vi "MOTOR CONTROL WITH PID AE.vi"(1 "Yaw":dbl, 2 "Speed":dbl, 3 "Direction":T1, 4 "AE Mode":T2) -> (0 "Speed & distance":T3)   [LabVIEW 2018]
uses:
  MOTOR CONTROL WITH PID AE DATA MODE TYPE DEF.ctl
  MOTOR CONTROL WITH PID AE DIRECTION TYPE DEF.ctl
  <vilib>/Studica/Studica Toolkit/Background/Mxp Selection.ctl
  <vilib>/addons/control/pid/pid.llb/PID (DBL).vi
  <vilib>/addons/control/pid/NI_PID_pid.lvlib
panel:
  out "Vx":dbl
  in  "error in (no error)":errorcluster
  out "M2":dbl
  out "M1":dbl
  out "M0":dbl
  out "S2":dbl
  out "S1":dbl
  out "error out":errorcluster
  out "S0":dbl
  out "M2 Distance":dbl
  out "M1 Distance":dbl
  out "M0 Distance":dbl
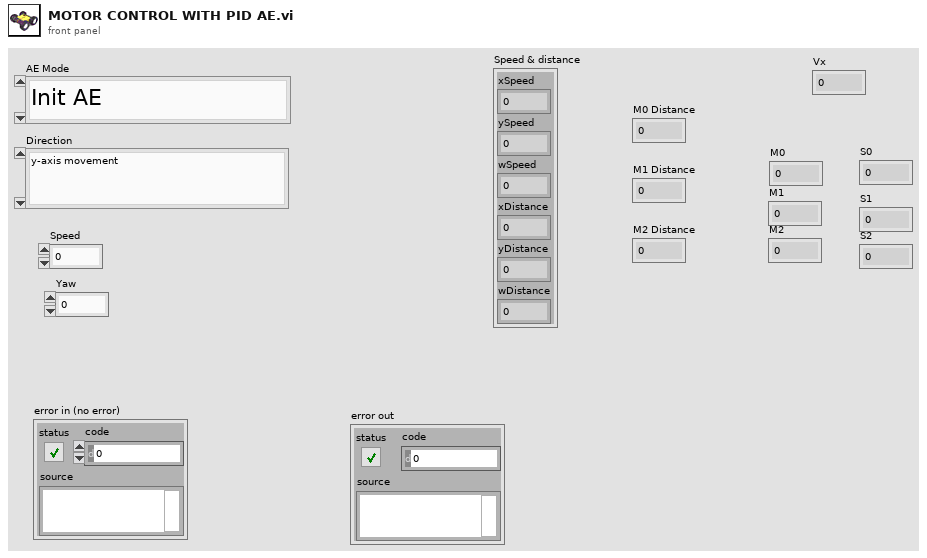
[diagram p1: front panel]
types:
  T1 = typedef "MOTOR CONTROL WITH PID AE DIRECTION TYPE DEF.ctl" = enum16{"y-axis movement", "x-axis movement", "rotation", "stop", "reset encoders"}
  T2 = typedef "MOTOR CONTROL WITH PID AE DATA MODE TYPE DEF.ctl" = enum16{"Init AE", "Write to AE", "Read from AE"}
  T3 = cluster{"xSpeed":dbl, "ySpeed":dbl, "wSpeed":dbl, "xDistance":dbl, "yDistance":dbl, "wDistance":dbl}
  T4 = cluster{"proportional gain (Kc)":dbl, "integral time (Ti, min)":dbl, "derivative time (Td, min)":dbl}
  T5 = typedef "Mxp Selection.ctl" = enum16{"MXP A", "MXP B"}
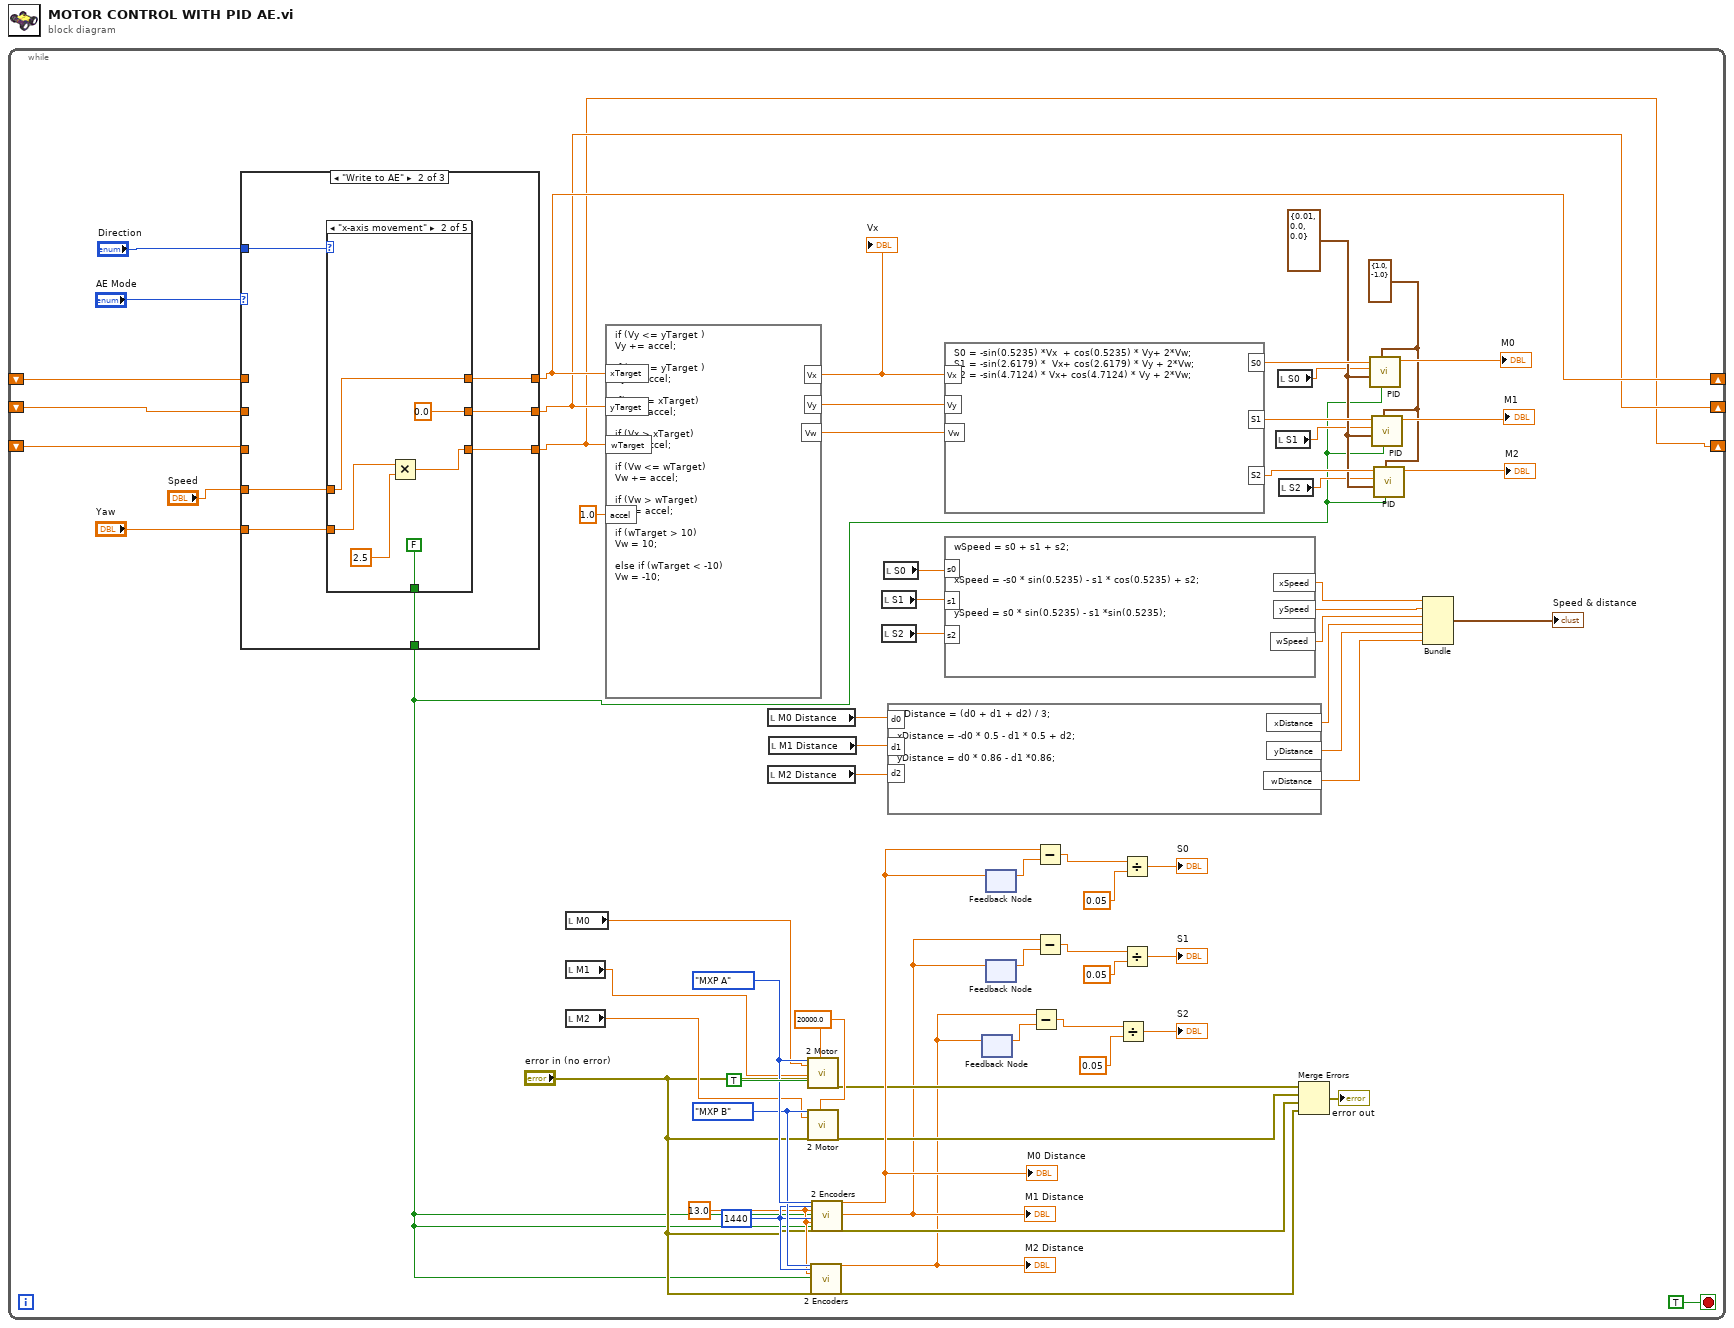
[diagram p0: block diagram]
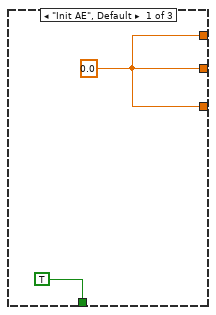
[diagram p2: hidden frame]
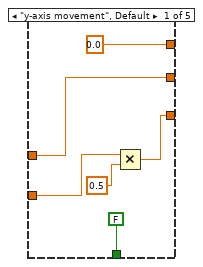
[diagram p3: hidden frame]
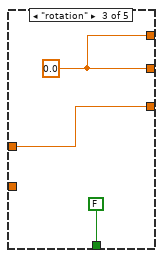
[diagram p4: hidden frame]
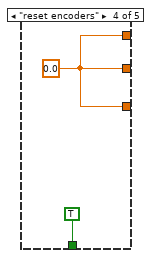
[diagram p5: hidden frame]
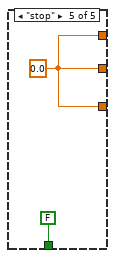
[diagram p6: hidden frame]
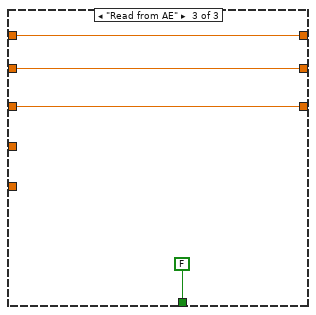
[diagram p7: hidden frame]
diagram:
  n1 = while {
    shift-right: [w9] -> _
    shift-left: _ -> [w12]
    shift-right: [w8] -> _
    shift-left: _ -> [w11]
    shift-right: [w7] -> _
    shift-left: _ -> [w10]
    stop <- TRUE stop-if-true
    w17 = T4 {"proportional gain (Kc)"=0.01, "integral time (Ti, min)"=0.0, "derivative time (Td, min)"=0.0} ("PID gains")
    w16 = cluster{"output high":dbl, "output low":dbl} {"output high"=1.0, "output low"=-1.0} ("output range")
    w65 = 13.0 ("Wheel Diameter M0 (inches)")
    w66 = u32 1440 ("Ticks Per Rev M0")
    w70 = 20000.0 ("Frequency [Hz]")
    w68 = Mxp_Selection."MXP A" ("Mxp Side")
    w67 = Mxp_Selection."MXP B" ("Mxp Side")
    n2 = case shown="\"Write to AE\"" "AE Mode" {
      tunnel: "Direction" -> [_ w79 _]
      tunnel: "Speed" -> [_ w78 _]
      tunnel: "Yaw" -> [_ w77 _]
      tunnel: [w72 w76 w101] -> w9
      tunnel: [w72 w75 w99] -> w7
      tunnel: [w72 w74 w100] -> w8
      tunnel: w12 -> [_ _ w101]
      tunnel: w11 -> [_ _ w100]
      tunnel: w10 -> [_ _ w99]
      tunnel: [TRUE w73 FALSE] -> w6
      frame "Init AE", Default {
        w72 = 0.0 ("input variable")
      }
      frame "Write to AE" {
        n3 = case shown="\"x-axis movement\"" w79 {
          tunnel: w78 -> [w85 w91 w94 _ _]
          tunnel: w77 -> [w82 w88 _ _ _]
          tunnel: [0.0 ("Speed") w91 w93 w96 w98] -> w76
          tunnel: [w81 w86 w94 w96 w98] -> w75
          tunnel: [w85 0.0 ("input variable") w93 w96 w98] -> w74
          tunnel: [FALSE FALSE FALSE TRUE FALSE] -> w73
          frame "y-axis movement", Default {
            n4 = Multiply(x=w82, y=0.5) -> (x*y=w81:dbl)
          }
          frame "x-axis movement" {
            n5 = Multiply(x=w88, y=2.5) -> (x*y=w86:dbl)
          }
          frame "rotation" {
            w93 = 0.0 ("input variable")
          }
          frame "reset encoders" {
            w96 = 0.0 ("input variable")
          }
          frame "stop" {
            w98 = 0.0 ("input variable")
          }
        }
      }
      frame "Read from AE" {
      }
    }
    n6 = local read "M0"() -> (w44:dbl)
    n7 = local read "M1"() -> (w43:dbl)
    n8 = local read "M2"() -> (w42:dbl)
    n9 = formula code="if (Vy <= yTarget )\nVy += accel;\n\nif (Vy >= yTarget )\nVy -= accel;\n\nif(Vx <= xTarget)\nVx += accel;\n\nif (Vx > xTarget)\nVx -= accel;\n\nif (Vw <= wTarget)\nVw += accel;\n\nif (Vw > wTarget)\nVw -= accel;\n\nif (wTarget > 10)\nVw = 10;\n\nelse if (wTarget < -10)\nVw = -10;"("xTarget"=w9, "yTarget"=w8, "wTarget"=w7, "accel"=1.0 ("input variable")) -> ("Vy"=w25:dbl, "Vx"=w26:dbl, "Vw"=w24:dbl)
    "Vx" <- w26
    n10 = local read "M0 Distance"() -> (w38:dbl)
    n11 = local read "M2 Distance"() -> (w36:dbl)
    n12 = local read "M1 Distance"() -> (w37:dbl)
    n13 = call <vilib>:"2 Motor.vi"("Mxp Side"=w68, "Speed M0"=w44, "Speed M1"=w43, "Invert M1"=TRUE, "error in (no error)"="error in (no error)", "Frequency [Hz]"=w70) -> ("error out"=w60:errorcluster)  [unwired: 13 in]
    n14 = call <vilib>:"2 Motor.vi"("Mxp Side"=w67, "Speed M0"=w42, "error in (no error)"="error in (no error)", "Frequency [Hz]"=w70) -> ("error out"=w59:errorcluster)  [unwired: 15 in]
    n15 = call <vilib>:"2 Encoders.vi"("Mxp Side"=w67, "Ticks Per Rev M0"=w66, "Wheel Diameter M0 (inches)"=w65, "Reset Encoder 0"=w6, "error in (no error)"="error in (no error)") -> ("Distance M0 (inches)"=w48:dbl, "error out"=w57:errorcluster)  [unwired: 20 in, 1 out]
    "M2 Distance" <- w48
    n16 = call <vilib>:"2 Encoders.vi"("Mxp Side"=w68, "Ticks Per Rev M0"=w66, "Wheel Diameter M0 (inches)"=w65, "Reset Encoder 0"=w6, "Ticks Per Rev M1"=w66, "Wheel Diameter M1 (inches)"=w65, "Reset Encoder 1"=w6, "error in (no error)"="error in (no error)") -> ("Distance M0 (inches)"=w63:dbl, "Distance M1 (inches)"=w52:dbl, "error out"=w58:errorcluster)  [unwired: 17 in]
    "M0 Distance" <- w63
    "M1 Distance" <- w52
    n17 = local read "S1"() -> (w40:dbl)
    n18 = local read "S2"() -> (w39:dbl)
    n19 = local read "S0"() -> (w41:dbl)
    n20 = formula code="wDistance = (d0 + d1 + d2) / 3;\n\nxDistance = -d0 * 0.5 - d1 * 0.5 + d2;\n\nyDistance = d0 * 0.86 - d1 *0.86;"("d0"=w38, "d1"=w37, "d2"=w36) -> ("xDistance"=w31:dbl, "wDistance"=w29:dbl, "yDistance"=w30:dbl)
    n21 = formula code="S0 = -sin(0.5235) *Vx  + cos(0.5235) * Vy+ 2*Vw;\nS1 = -sin(2.6179) *  Vx+ cos(2.6179) * Vy + 2*Vw;\nS2 = -sin(4.7124) * Vx+ cos(4.7124) * Vy + 2*Vw;"("Vx"=w26, "Vy"=w25, "Vw"=w24) -> ("S0"=w23:dbl, "S1"=w22:dbl, "S2"=w21:dbl)
    n22 = formula code="wSpeed = s0 + s1 + s2;\n\n\nxSpeed = -s0 * sin(0.5235) - s1 * cos(0.5235) + s2;\n\n\nySpeed = s0 * sin(0.5235) - s1 *sin(0.5235);"("s0"=w41, "s1"=w40, "s2"=w39) -> ("xSpeed"=w35:dbl, "ySpeed"=w34:dbl, "wSpeed"=w33:dbl)
    n23 = feedback #1() -> (w50:dbl)  [unwired: 1 in]
    n24 = feedback-in #1(w48) -> ()
    n25 = feedback #2() -> (w62:dbl)  [unwired: 1 in]
    n26 = feedback-in #2(w63) -> ()
    n27 = feedback #3() -> (w54:dbl)  [unwired: 1 in]
    n28 = feedback-in #3(w52) -> ()
    n29 = Subtract(x=w48, y=w50) -> (x-y=w51:dbl)
    n30 = Subtract(x=w63, y=w62) -> (x-y=w64:dbl)
    n31 = Subtract(x=w52, y=w54) -> (x-y=w55:dbl)
    n32 = Divide(x=w51, y=0.05) -> (x/y=→"S2":dbl)
    n33 = Divide(x=w64, y=0.05) -> (x/y=→"S0":dbl)
    n34 = Divide(x=w55, y=0.05) -> (x/y=→"S1":dbl)
    n35 = local read "S1"() -> (w14:dbl)
    n36 = local read "S0"() -> (w15:dbl)
    n37 = local read "S2"() -> (w13:dbl)
    n38 = Merge Errors(w60, w59, w58, w57) -> (→"error out":errorcluster)
    n39 = call-poly <vilib>:"PID.vi"("reinitialize? (F)"=w6, "output range"=w16, "PID gains"=w17, "process variable"=w15, "setpoint"=w23) -> ("output"=→"M0":dbl)  [unwired: 5 in, 1 out]
    n40 = call-poly <vilib>:"PID.vi"("reinitialize? (F)"=w6, "output range"=w16, "PID gains"=w17, "process variable"=w14, "setpoint"=w22) -> ("output"=→"M1":dbl)  [unwired: 5 in, 1 out]
    n41 = call-poly <vilib>:"PID.vi"("reinitialize? (F)"=w6, "output range"=w16, "PID gains"=w17, "process variable"=w13, "setpoint"=w21) -> ("output"=→"M2":dbl)  [unwired: 5 in, 1 out]
    n42 = Bundle("xSpeed"=w35, "ySpeed"=w34, "wSpeed"=w33, "xDistance"=w31, "yDistance"=w30, "wDistance"=w29) -> (→"Speed & distance":T3)  [unwired: 1 in]
  }
